vi "Finish.vi"   [LabVIEW 2018]
doc: "This VI is called just before exiting. It is expected to close I/O refnum, save collected data, etc."
uses:
  <vilib>/Rock Robotics/WPI/Utilities/WPI_GetSetVariantRefNum.vi
types:
  T1 = typedef "WPI_JoystickDevRef.ctl" = cluster{"Device":T2}
  T2 = typedef "WPI_JoystickDeviceEnum.ctl" = enum16{"USB 0", "USB 1", "USB 2", "USB 3", "USB 4", "USB 5"}
  T3 = typedef "WPI_DigitalInputDevRef.ctl" = cluster{"DevStatus":errorcluster, "DIO Channel":T4}
  T4 = typedef "FPGA_DIOChannel.ctl" = enum8{"DIO 0", "DIO 1", "DIO 2", "DIO 3", "DIO 4", "DIO 5", "DIO 6", "DIO 7", "DIO 8", "DIO 9", "DIO MXP 0", "DIO MXP 1", "DIO MXP 2", "DIO MXP 3", "DIO MXP 4", "DIO MXP 5", "DIO MXP 6", "DIO MXP 7", "DIO MXP 8", "DIO MXP 9", "DIO MXP 10", "DIO MXP 11", "DIO MXP 12", "DIO MXP 13", "DIO MXP 14", "DIO MXP 15", "SPI Port CS1", "SPI Port CS2", "SPI Port CS3", "SPI Port MISO", "SPI Port MOSI", "Invalid"}
  T5 = typedef "WPI_SolenoidDevRef.ctl" = cluster{"DevStatus":errorcluster, "Pneumatics Control Module":u8, "Forward Solenoid Channel":T6, "Reverse Solenoid Channel":T6}
  T6 = typedef "WPI_SolenoidChannel.ctl" = enum8{"Solenoid 0", "Solenoid 1", "Solenoid 2", "Solenoid 3", "Solenoid 4", "Solenoid 5", "Solenoid 6", "Solenoid 7", "Invalid"}
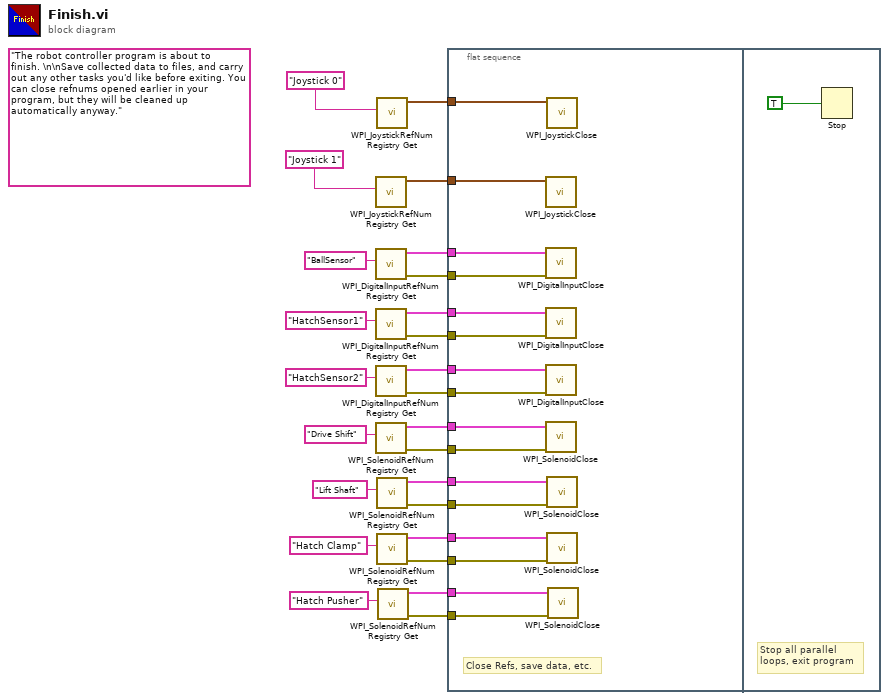
[diagram p0: block diagram]
diagram:
  (unwired) "The robot controller program is about to finish. \n\nSave collected data to files, and carry out any other tasks you'd like before exiting. You can close refnums opened earlier in your program, but they will be cleaned up automatically anyway."
  n1 = call <vilib>:"WPI_JoystickRefNum Registry Get.vi"("refnum name"="Joystick 1") -> ("JoystickDevRef"=w23:T1)  [unwired: 1 in, 9 out]
  n2 = call <vilib>:"WPI_DigitalInputRefNum Registry Get.vi"("refnum name"="BallSensor") -> ("error out"=w20:errorcluster, "DigitalInputDevRef"=w21:T3)  [unwired: 9 in]
  n3 = call <vilib>:"WPI_DigitalInputRefNum Registry Get.vi"("refnum name"="HatchSensor1") -> ("error out"=w17:errorcluster, "DigitalInputDevRef"=w16:T3)  [unwired: 9 in]
  n4 = call <vilib>:"WPI_DigitalInputRefNum Registry Get.vi"("refnum name"="HatchSensor2") -> ("error out"=w14:errorcluster, "DigitalInputDevRef"=w15:T3)  [unwired: 9 in]
  n5 = call <vilib>:"WPI_SolenoidRefNum Registry Get.vi"("refnum name"="Drive Shift") -> ("error out"=w11:errorcluster, "SolenoidDevRef"=w12:T5)  [unwired: 9 in]
  n6 = call <vilib>:"WPI_JoystickRefNum Registry Get.vi"("refnum name"="Joystick 0") -> ("JoystickDevRef"=w24:T1)  [unwired: 1 in, 9 out]
  n7 = call <vilib>:"WPI_SolenoidRefNum Registry Get.vi"("refnum name"="Lift Shaft") -> ("error out"=w8:errorcluster, "SolenoidDevRef"=w7:T5)  [unwired: 9 in]
  n8 = call <vilib>:"WPI_SolenoidRefNum Registry Get.vi"("refnum name"="Hatch Clamp") -> ("error out"=w5:errorcluster, "SolenoidDevRef"=w6:T5)  [unwired: 9 in]
  n9 = call <vilib>:"WPI_SolenoidRefNum Registry Get.vi"("refnum name"="Hatch Pusher") -> ("error out"=w2:errorcluster, "SolenoidDevRef"=w1:T5)  [unwired: 9 in]
  n10 = flat-sequence {
    tunnel: w24 -> [w41]
    tunnel: w23 -> [w40]
    tunnel: w21 -> [w39]
    tunnel: w20 -> [w38]
    tunnel: w16 -> [w36]
    tunnel: w17 -> [w37]
    tunnel: w15 -> [w35]
    tunnel: w14 -> [w34]
    tunnel: w12 -> [w33]
    tunnel: w11 -> [w32]
    tunnel: w7 -> [w30]
    tunnel: w8 -> [w31]
    tunnel: w6 -> [w29]
    tunnel: w5 -> [w28]
    tunnel: w1 -> [w26]
    tunnel: w2 -> [w27]
    frame #0 {
      # "Close Refs, save data, etc."
      n11 = call <vilib>:"WPI_JoystickClose.vi"("JoystickDevRef"=w40) -> ()  [unwired: 11 out]
      n12 = call <vilib>:"WPI_DigitalInputClose.vi"("error in (no error)"=w38, "DigitalInputDevRef"=w39) -> ()  [unwired: 9 in, 1 out]
      n13 = call <vilib>:"WPI_DigitalInputClose.vi"("error in (no error)"=w37, "DigitalInputDevRef"=w36) -> ()  [unwired: 9 in, 1 out]
      n14 = call <vilib>:"WPI_DigitalInputClose.vi"("error in (no error)"=w34, "DigitalInputDevRef"=w35) -> ()  [unwired: 9 in, 1 out]
      n15 = call <vilib>:"WPI_SolenoidClose.vi"("error in (no error)"=w32, "SolenoidDevRef"=w33) -> ()  [unwired: 9 in, 1 out]
      n16 = call <vilib>:"WPI_JoystickClose.vi"("JoystickDevRef"=w41) -> ()  [unwired: 11 out]
      n17 = call <vilib>:"WPI_SolenoidClose.vi"("error in (no error)"=w31, "SolenoidDevRef"=w30) -> ()  [unwired: 9 in, 1 out]
      n18 = call <vilib>:"WPI_SolenoidClose.vi"("error in (no error)"=w28, "SolenoidDevRef"=w29) -> ()  [unwired: 9 in, 1 out]
      n19 = call <vilib>:"WPI_SolenoidClose.vi"("error in (no error)"=w27, "SolenoidDevRef"=w26) -> ()  [unwired: 9 in, 1 out]
    }
    frame #1 {
      # "Stop all parallel\nloops, exit program"
      n20 = Stop(stop? (T)=TRUE ("Quit")) -> ()
    }
  }
